vi "HowToChangeRegime.vi"(10 "Desired Sailing Regime":T1, 11 "Current Sailing Regime":T1) -> (3 "Output sailing regime":T1)   [LabVIEW 2013]
doc: "This VI looks at the regime that the boat is in and the desired regime, then determines how best to get there from the current position. This code will only ever increment and decrement the regime by one state, so to go in a circle the boat must step from one state to the other. This is done on purpose as part of the MB structure.\n\nFor example, if we are on a port tack and want to be on a starboard tack, this VI should tell the boat to tack to port. If the boat needs to go from starboard tack to close to running with the wind over the starboard bow, this VI should tell the boat to go into the 'Turn w/o crossing wind' behavior, to port.\n\nThis shouldn't get either transitions as inputs or two of the same regime as an input, because it's within case structures that prevent those two types of inputs from coming in. If those outer case statements get changes, rexamine the effect on this code.\n\nEric Schneider, Feb. 2014"
uses:
  Data/TypeDefs/Sailing Regimes.ctl
panel:
  out "Suggested regime modification":i32
  out "Difference\nbetween\nregimes":u16
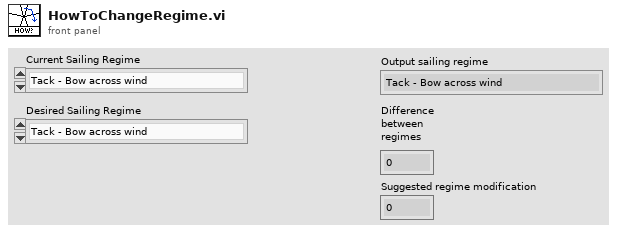
[diagram p1: front panel]
types:
  T1 = typedef "Sailing Regimes.ctl" = enum16{"Tack - Bow across wind", "Upwind - Starboard Tack", "Turn between Upwind/Reach - Starboard Tack", "Reach - Starboard Tack", "Turn between Reach/Run - Starboard Tack", "Run - Starboard Tack", "Jibe - Stern across wind", "Run - Port Tack", "Turn between Reach/Run - Port Tack", "Reach - Port Tack", "Turn between Upwind/Reach - Port Tack", "Upwind - Port Tack"}
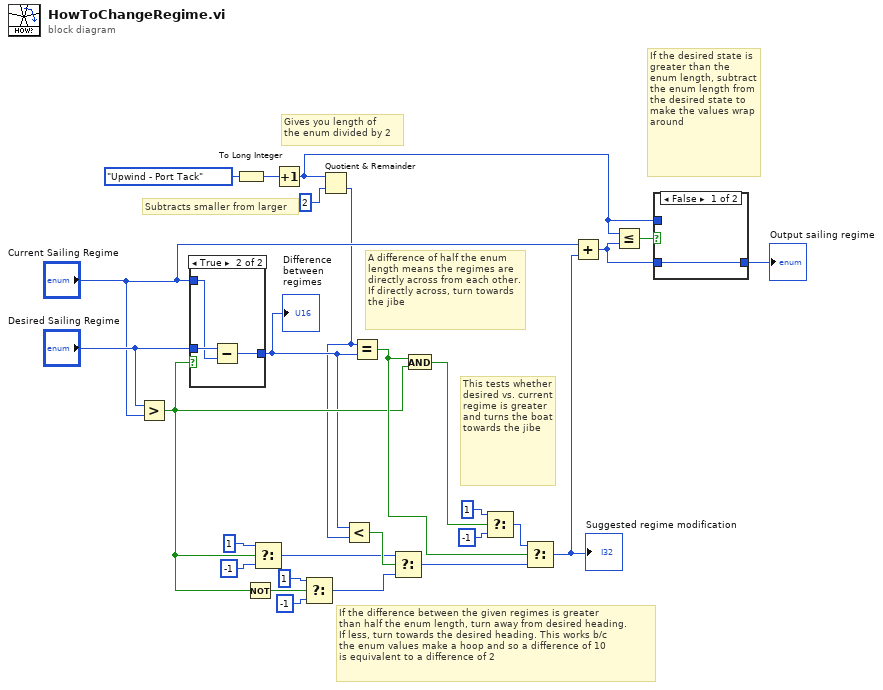
[diagram p0: block diagram]
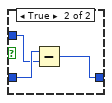
[diagram p2: hidden frame]
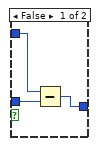
[diagram p3: hidden frame]
diagram:
  # "If the desired state is greater than the enum length, subtract the enum length from the desired state to make the values wrap around"
  # "If the difference between the given regimes is greater\nthan half the enum length, turn away from desired heading.\nIf less, turn towards the desired heading. This works b/c\nthe enum values make a hoop and so a difference of 10\nis equivalent to a difference of 2"
  # "Gives you length of\nthe enum divided by 2"
  # "This tests whether desired vs. current regime is greater and turns the boat towards the jibe"
  # "A difference of half the enum length means the regimes are directly across from each other. If directly across, turn towards the jibe"
  # "Subtracts smaller from larger"
  n1 = Greater?(x="Desired Sailing Regime", y="Current Sailing Regime") -> (0:w11:bool)
  n2 = case shown="True" w11 {
    tunnel: "Desired Sailing Regime" -> [w30 w33]
    tunnel: "Current Sailing Regime" -> [w29 w32]
    tunnel: [w28 w31] -> w6
    frame False {
      n3 = Subtract(x=w29, y=w30) -> (x-y=w28:u16)
    }
    frame True {
      n4 = Subtract(x=w33, y=w32) -> (x-y=w31:u16)
    }
  }
  "Difference\nbetween\nregimes" <- w6
  n5 = To Long Integer(number=Sailing_Regimes."Upwind - Port Tack" ("Desired Sailing Regime")) -> (32bit integer=w8:i32)
  n6 = Not(x=w11) -> (.not. x?=w12:bool)
  n7 = Select(t=1, s=w11, f=-1) -> (s? t:f=w15:i32)
  n8 = Increment(x=w8) -> (x+1=w1:i32)
  n9 = Select(t=1, s=w12, f=-1) -> (s? t:f=w10:i32)
  n10 = Quotient & Remainder(x=w1, y=2) -> (floor(x/y)=w5:i32)  [unwired: 1 out]
  n11 = Less?(x=w6, y=w5) -> (x < y?=w19:bool)
  n12 = Equal?(x=w5, y=w6) -> (x = y?=w23:bool)
  n13 = Select(t=w15, s=w19, f=w10) -> (s? t:f=w18:i32)
  n14 = And(x=w23, y=w11) -> (x .and. y?=w26:bool)
  n15 = Select(t=1, s=w26, f=-1) -> (s? t:f=w22:i32)
  n16 = Select(t=w22, s=w23, f=w18) -> (s? t:f=w20:i32)
  "Suggested regime modification" <- w20
  n17 = Add(x="Current Sailing Regime", y=w20) -> (x+y=w3:i32)
  n18 = Less Or Equal?(x=w1, y=w3) -> (x <= y?=w4:bool)
  n19 = case shown="False" w4 {
    tunnel: w3 -> [w34 w37]
    tunnel: [w34 w35] -> w2
    tunnel: w1 -> [_ w36]
    frame False {
    }
    frame True {
      n20 = Subtract(x=w37, y=w36) -> (x-y=w35:i32)
    }
  }
  "Output sailing regime" <- w2
